vi "position.vi"() -> ()   [LabVIEW 2013]
panel:
  out "Position":dbl[](array[numeric]) format="%.6f"
  in  "error in":errorcluster
  out "Conn. Axes":string[](array[string])
  out "Identification":string
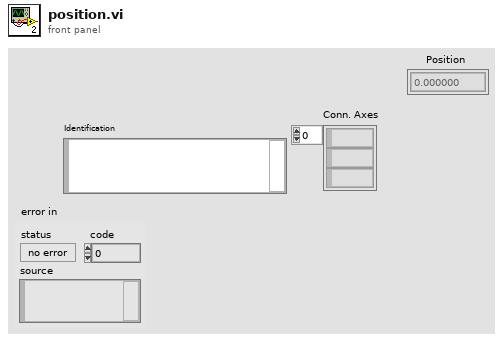
[diagram p1: front panel]
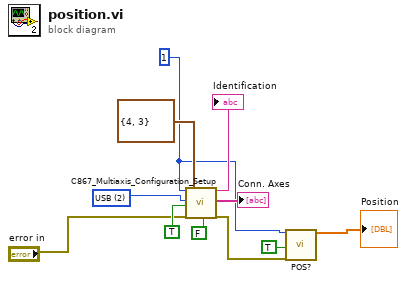
[diagram p0: block diagram]
diagram:
  w7 = u16 2 items=["RS232", "RS232 DaisyChain", "USB"] ("Interface")
  w4 = 1 ("System no.")
  n1 = call "C867_Multiaxis_Configuration_Setup.vi"("System no."=w4, "Interface"=w7, "All axes?"=TRUE, "error in"="error in", "RS232 settings"=cluster{"Portnumber":i32, "Baudrate":u16} {"Portnumber"=4, "Baudrate"=3}, "Switch servo on?"=FALSE ("Use dialog to define\nconnected stages?")) -> ("Identification"=→"Identification":string, "Conn. \nAxes"=→"Conn. Axes":string[], "error out"=w3:errorcluster)  [unwired: 7 in, 4 out]
  n2 = call "POS?.vi"("System no."=w4, "All axes?"=TRUE, "error in"=w3) -> ("Position"=→"Position":dbl[])  [unwired: 15 in, 1 out]
